vi "Make path.vi"(10 "what?":string="opimisation file", 11 "name":string) -> (3 "path":path)   [LabVIEW 2012, in "RSA.lvclass"]
uses:
  RSA.lvclass
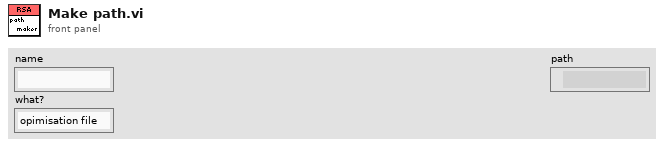
[diagram p1: front panel]
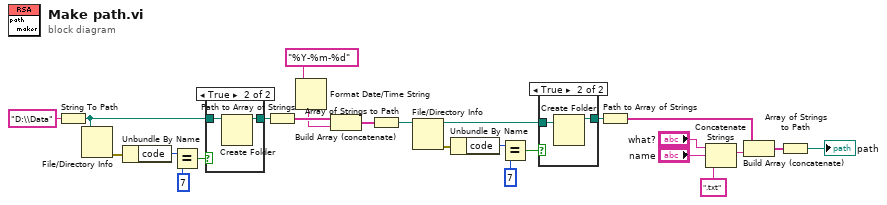
[diagram p0: block diagram]
diagram:
  n1 = String To Path(string="D:\\Data") -> (path=w20:path)
  n2 = File/Directory Info(path=w20) -> (error out=w24:errorcluster)  [unwired: 1 in, 6 out]
  n3 = Unbundle By Name(w24) -> ("code"=w23:i32)
  n4 = Equal?(x=w23, y=7) -> (x = y?=w21:bool)
  n5 = case shown="True" w21 {
    tunnel: w20 -> [w26 w28]
    tunnel: [w26 w27] -> w18
    frame False {
    }
    frame True {
      n6 = Create Folder(path (use dialog)=w28) -> (created path=w27:path)  [unwired: 1 in, 3 out]
    }
  }
  n7 = Path to Array of Strings(0:w18) -> (2:w16:string[])  [unwired: 1 out]
  n8 = Format Date/Time String(time format string (%c)="%Y-%m-%d") -> (date/time string=w15:string)  [unwired: 2 out]
  n9 = Build Array (concatenate)(w16, w15) -> (w14:string[])
  n10 = Array of Strings to Path(0:w14) -> (2:w12:path)  [unwired: 1 out]
  n11 = File/Directory Info(path=w12) -> (path out=w8:path, error out=w11:errorcluster)  [unwired: 1 in, 5 out]
  n12 = Unbundle By Name(w11) -> ("code"=w10:i32)
  n13 = Equal?(x=w10, y=7) -> (x = y?=w9:bool)
  n14 = case shown="True" w9 {
    tunnel: w8 -> [w29 w31]
    tunnel: [w29 w30] -> w3
    frame False {
    }
    frame True {
      n15 = Create Folder(path (use dialog)=w31) -> (created path=w30:path)  [unwired: 1 in, 3 out]
    }
  }
  n16 = Path to Array of Strings(0:w3) -> (2:w7:string[])  [unwired: 1 out]
  n17 = Concatenate Strings("what?", "name", ".txt" ("string")) -> (w6:string)
  n18 = Build Array (concatenate)(w7, w6) -> (w5:string[])
  n19 = Array of Strings to Path(0:w5) -> (2:→"path":path)  [unwired: 1 in]
